vi "Read Address Bus.vi"(8 "error in (no error)":errorcluster, 11 "IO in":refnum<class "IO.lvclass">) -> (0 "error out":errorcluster, 3 "IO out":refnum<class "IO.lvclass">)   [LabVIEW 2021, in "IO.lvclass"]
uses:
  IO.lvclass
  IO.lvclass/IO.ctl
  <vilib>/DAQmx/read.llb/DAQmx Read (Digital 1D Bool NChan 1Samp 1Line).vi
  <vilib>/DAQmx/miscellaneous.llb/DAQmx Fill In Error Info.vi
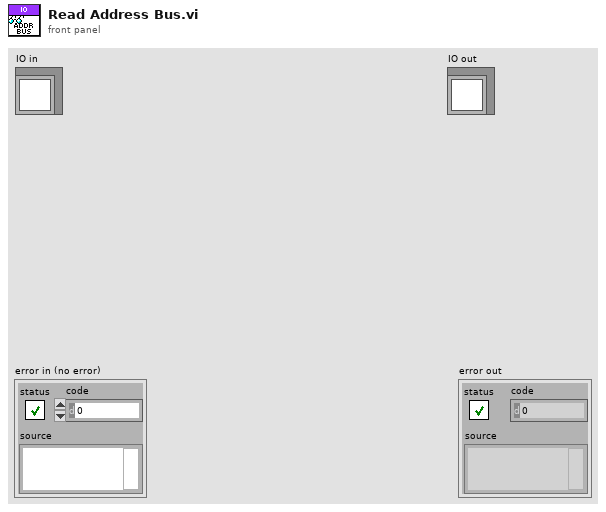
[diagram p1: front panel]
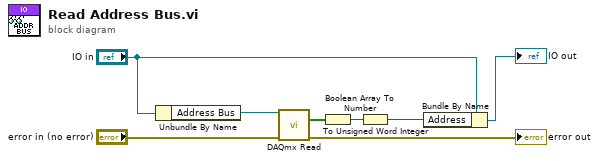
[diagram p0: block diagram]
diagram:
  n1 = Unbundle By Name("IO in") -> ("Address Bus"=w6:refnum<k21>)
  n2 = call-poly <vilib>:"DAQmx Read.vi"("task/channels in"=w6, "error in"="error in (no error)") -> ("data"=w4:bool[], "error out"=→"error out":errorcluster)  [unwired: 11 in, 1 out]
  n3 = Boolean Array To Number(Boolean array=w4) -> (number=w5:u32)
  n4 = To Unsigned Word Integer(number=w5) -> (unsigned 16bit integer=w2:u16)
  n5 = Bundle By Name(cluster="IO in", "Address"=w2) -> (→"IO out":refnum<class "IO.lvclass">)
